vi "Get Instrument Info.vi"(0 "Simulated Power Meter in":refnum<class "Simulated Power Meter.lvclass">, 11 "error in":errorcluster) -> (4 "Simulated Power Meter out":refnum<class "Simulated Power Meter.lvclass">, 15 "error out":errorcluster)   [LabVIEW 2023, in "RFFixtureCharact.Instruments.lvlib" / "Simulated Power Meter.lvclass"]
uses:
  Simulated Power Meter.lvclass
  C:/srd-semi-rfcal-software/AuxTools/STSRFFixtureCharactUtility/Source/Code Modules/Fixture/Instruments/Power Meter/Power Meter Base/Power Meter Base.lvclass
  Power Meter Base/Type Definitions/Instrument Info.ctl
  Power Meter Base/Power Meter Base.lvclass/Power Meter Base.ctl
  Power Meter Base/Properties/Write Instrument Info Array.vi
  Common/Data Cache/Settings Dictionary/Setting Keys.vi
  Common/RFCalAndFixtureCharact.Common.lvlib
  Power Meter Base/Power Meter Base.lvclass
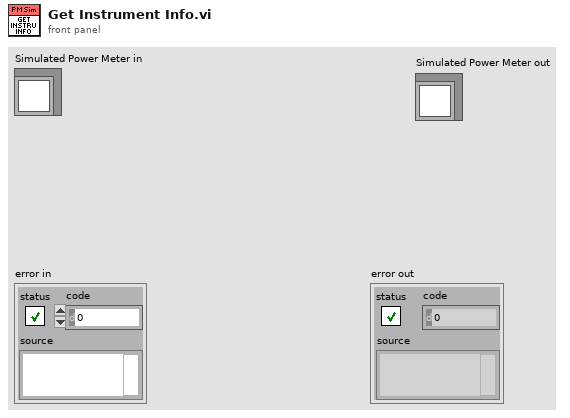
[diagram p1: front panel]
types:
  T1 = typedef "RFFixtureCharact.Instruments.lvlib/Power Meter Base.lvclass/Instrument Info.ctl" = cluster{"User Alias":string, "Resource Name":string, "Product Name":string, "Vendor Name":string}
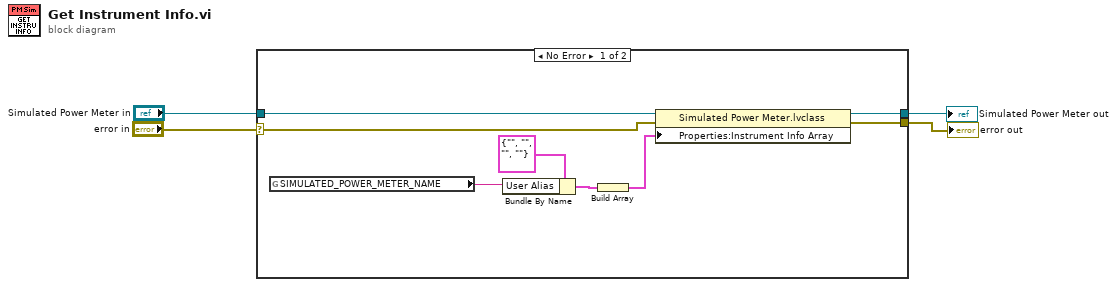
[diagram p0: block diagram]
diagram:
  n1 = case shown="No Error" "error in" {
    selector: "error in" -> [w10 w13]
    tunnel: [w9 w13] -> w3
    tunnel: [w11 w14] -> w1
    tunnel: "Simulated Power Meter in" -> [w12 w14]
    frame No Error {
      n2 = global read "Setting Keys.vi" "SIMULATED_POWER_METER_NAME"() -> (w7:string)
      n3 = Bundle By Name(cluster=T1 {"User Alias"="", "Resource Name"="", "Product Name"="", "Vendor Name"=""} ("Instrument Info Cluster"), "User Alias"=w7) -> (w6:T1)
      n4 = Build Array(w6) -> (w5:T1[])
      n5 = property class="Simulated Power Meter.lvclass"(reference=w12, error in=w10, "Properties:Instrument Info Array"=w5) -> (reference out=w11:refnum<class "Simulated Power Meter.lvclass">, error out=w9:errorcluster)
    }
    frame Error {
    }
  }
  "error out" <- w3
  "Simulated Power Meter out" <- w1
